vi "Auto Fit Width By Col.vi"(8 "error in (no error)":errorcluster caption="错误输入（无错误）", 11 "Table Ref In":refnum<vi>) -> (0 "error out":errorcluster caption="错误输出", 3 "Table Ref Out":refnum<vi>)   [LabVIEW 2012, in "Table Tool.lvlib"]
uses:
  Table Tool.lvlib
  <vilib>/Utility/miscctls.llb/LVRowAndColumnTypeDef.ctl
  Property/Set Or Get Value.vi
panel:
  in  "Space":i16=20
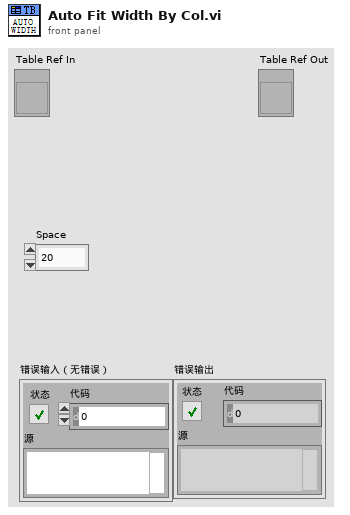
[diagram p1: front panel]
types:
  T1 = typedef "LVRowAndColumnTypeDef.ctl" = cluster{"Row":i32, "Column":i32}
  T2 = cluster{"left":i16, "top":i16, "right":i16, "bottom":i16}
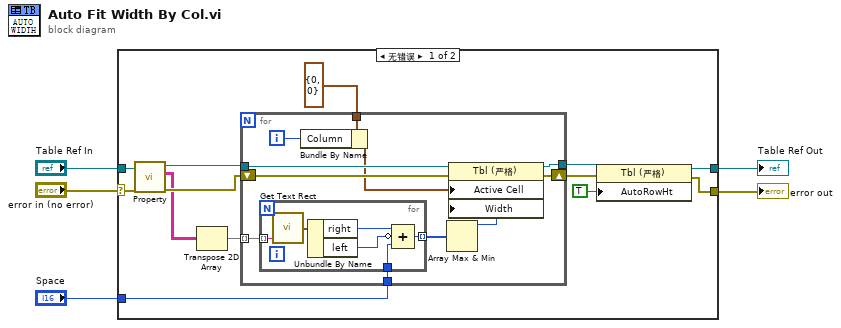
[diagram p0: block diagram]
diagram:
  n1 = case shown="无错误" "error in (no error)" {
    selector: "error in (no error)" -> [w17 w37]
    tunnel: "Table Ref In" -> [w18 w36]
    tunnel: [w10 w36] -> w3
    tunnel: [w9 w37] -> w2
    tunnel: "Space" -> [w16 _]
    frame No Error {
      n2 = call-poly "Property.vi"("error in (no error)"=w17, "Table Ref In"=w18) -> ("error out"=w14:errorcluster, "Value Out"=w7:string[][], "Table Ref Out"=w15:refnum<vi>)  [unwired: 7 in]
      n3 = Transpose 2D Array(2D array=w7) -> (transposed array=w6:string[][])
      n4 = for {
        tunnel: w16 -> [w29]
        tunnel: w15 -> [w26]
        shift-right: [w27] -> w12
        shift-left: w14 -> [w28]
        tunnel: [w25] -> w13
        tunnel: T1 {"Row"=0, "Column"=0} ("Active Cell:Active Cell") -> [w24]
        tunnel: w6 -> [w21] mode=indexing
        i -> [w23]
        n5 = for {
          tunnel: w29 -> [w32]
          tunnel: [w31] -> w20 mode=indexing
          tunnel: w21 -> [w30] mode=indexing
          n6 = call <vilib>:"Get Text Rect.vi"("text"=w30) -> ("rect"=w35:T2)  [unwired: 8 in]
          n7 = Unbundle By Name(w35) -> ("right"=w34:i16, "left"=w33:i16)
          n8 = Compound Arithmetic op=ADD(w34, invert w33, w32) -> (w31:i16)
        }
        n9 = Bundle By Name(cluster=w24, "Column"=w23) -> (w22:T1)
        n10 = Array Max & Min(array=w20) -> (max value=w19:i16)  [unwired: 3 out]
        n11 = property class="Tbl (严格)"(reference=w26, error in=w28, "Active Cell"=w22, "Width"=w19) -> (reference out=w25:refnum<vi>, error out=w27:errorcluster)
      }
      n12 = property class="Tbl (严格)"(reference=w13, error in=w12, "AutoRowHt"=TRUE ("自动调整行高")) -> (reference out=w10:refnum<vi>, error out=w9:errorcluster)
    }
    frame Error {
    }
  }
  "Table Ref Out" <- w3
  "error out" <- w2
